vi "Update DAQmx Finite Task.vi"(8 "error in (no error)":errorcluster, 10 "measurement configuration":T1={"digital channel list"="", "frame clock rate"=0.0, "number of channels"=0, "channel length"=0, "bit depth"=0, "data justification"=enum."Left Justified", "endianness"=enum."MSB First", "bit clock edge sync"=enum."Rising", "frame sync edge for channel 0"=enum."Rising", "channel 0 offset"=0, "master clock channel list"="", "master clock rate"=0.0, "enable dither"=FALSE, "logic level"=enum."3.3 V", "signal frequency"=1000.0, "output level"=0.0, "output level units"=enum."% FS", "output range (pk-pk)"=0.0, "load impedance"=0.0, "signal phase"=0.0, "acq sampling rate"=0.0, "min measurement cycles"=0, "min measurement time (s)"=0.0, "min settling cycles"=0, "min settling time (s)"=0.0, "acq channel"="", "band start"=0.0, "band stop"=0.0, "weighting filter"=enum."Linear", "highpass filter"=enum."DC", "lowpass filter"=enum."No filter", "SNR units"=enum."dB", "THD+N units"=enum."dB", "THD units"=enum."dB", "gain units"=enum."dB"} {"signal phase" format="%0.2f"; "master clock rate" format="%#_6pHz"; "frame clock rate" format="%#_6pHz"}, 11 "task/channels in":refnum<k21>) -> (0 "error out":errorcluster, 3 "task out":refnum<k21>)   [LabVIEW 2022 SP3]
uses:
  controls/single tone measurement settings (HW).ctl
  controls/digital audio protocol/data justification.ctl
  controls/digital audio protocol/endianness.ctl
  controls/digital audio protocol/digital edge.ctl
  controls/digital audio protocol/logic level.ctl
  controls/digital output level units.ctl
  controls/weighting filter.ctl
  controls/highpass filter.ctl
  controls/lowpass filter.ctl
  controls/units - snr.ctl
  controls/units - ratio.ctl
  <vilib>/DAQmx/configure/timing.llb/DAQmx Timing (Sample Clock).vi
  controls/audio controls.lvlib
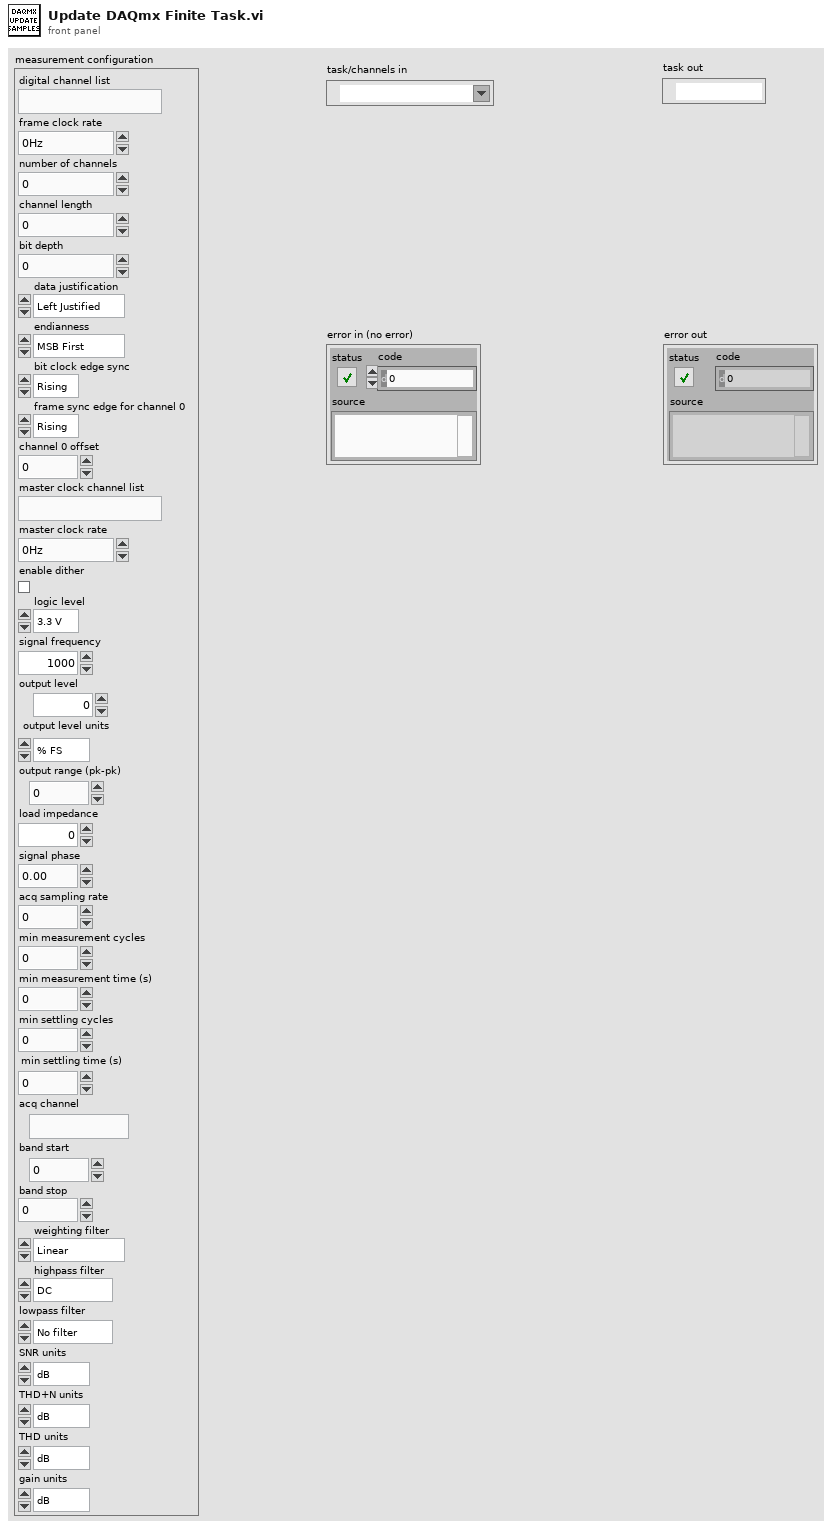
[diagram p1: front panel]
types:
  T1 = typedef "single tone measurement settings (HW).ctl" = cluster{"digital channel list":string, "frame clock rate":dbl, "number of channels":u32, "channel length":u32, "bit depth":u32, "data justification":T2, "endianness":T3, "bit clock edge sync":T4, "frame sync edge for channel 0":T4, "channel 0 offset":u32, "master clock channel list":string, "master clock rate":dbl, "enable dither":bool, "logic level":T5, "signal frequency":dbl, "output level":dbl, "output level units":T6, "output range (pk-pk)":dbl, "load impedance":dbl, "signal phase":dbl, "acq sampling rate":dbl, "min measurement cycles":u32, "min measurement time (s)":dbl, "min settling cycles":u32, "min settling time (s)":dbl, "acq channel":string, "band start":dbl, "band stop":dbl, "weighting filter":T7, "highpass filter":T8, "lowpass filter":T9, "SNR units":T10, "THD+N units":T11, "THD units":T11, "gain units":T11}
  T2 = typedef "data justification.ctl" = enum32{"Left Justified", "Right Justified"}
  T3 = typedef "endianness.ctl" = enum32{"MSB First", "LSB First"}
  T4 = typedef "digital edge.ctl" = enum32{"Rising", "Falling"}
  T5 = typedef "logic level.ctl" = enum32{"3.3 V", "1.8 V", "1.2 V"}
  T6 = typedef "audio controls.lvlib/digital output level units.ctl" = enum32{"% FS", "dBFS", "V"}
  T7 = typedef "weighting filter.ctl" = enum32{"Linear", "A-weighting", "B-weighting", "C-weighting"}
  T8 = typedef "highpass filter.ctl" = enum32{"DC", "AC"}
  T9 = typedef "lowpass filter.ctl" = enum32{"No filter", "AES17 20kHz", "AES17 40kHz"}
  T10 = typedef "audio controls.lvlib/units - snr.ctl" = enum32{"dB", "x/y"}
  T11 = typedef "audio controls.lvlib/units - ratio.ctl" = enum32{"dB", "%", "x/y"}
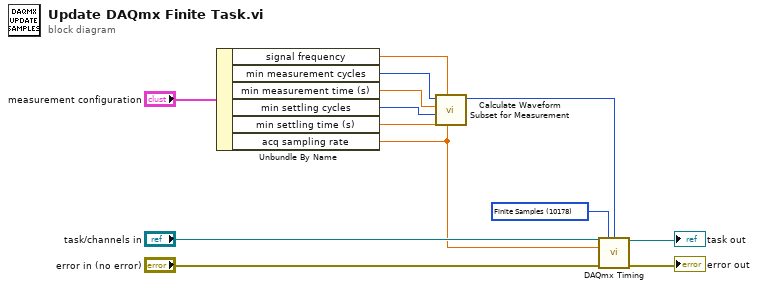
[diagram p0: block diagram]
diagram:
  w4 = 10178 items=["Finite Samples"=10178, "Continuous Samples"=10123, "Hardware Timed Single Point"=12522] ("sample mode")
  n1 = Unbundle By Name("measurement configuration") -> ("signal frequency"=w2:dbl, "min measurement cycles"=w9:u32, "min measurement time (s)"=w8:dbl, "min settling cycles"=w7:u32, "min settling time (s)"=w6:dbl, "acq sampling rate"=w3:dbl)
  n2 = call "Calculate Waveform Subset for Measurement.vi"("sampling rate"=w3, "signal frequency"=w2, "minimum settling duration"=w6, "minimum settling cycles"=w7, "minimum measurement duration"=w8, "minimum measurement cycles"=w9) -> ("total acquisition (samples)"=w5:u32)  [unwired: 3 in, 2 out]
  n3 = call-poly <vilib>:"DAQmx Timing.vi"("task/channels in"="task/channels in", "sample mode"=w4, "samples per channel"=w5, "rate"=w3, "error in"="error in (no error)") -> ("task out"=→"task out":refnum<k21>, "error out"=→"error out":errorcluster)  [unwired: 9 in]
